vi "Toggle Output(U64).vi"(6 "Iteration Count":u64=1000, 7 "reset(F)":bool) -> (2 "Signal":bool)   [LabVIEW 2017]
doc: "Toggles the Signal output every time the iteration count reaches the configured period. Wire reset(F) to restart the toggle period."
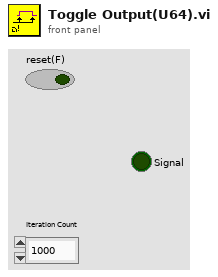
[diagram p1: front panel]
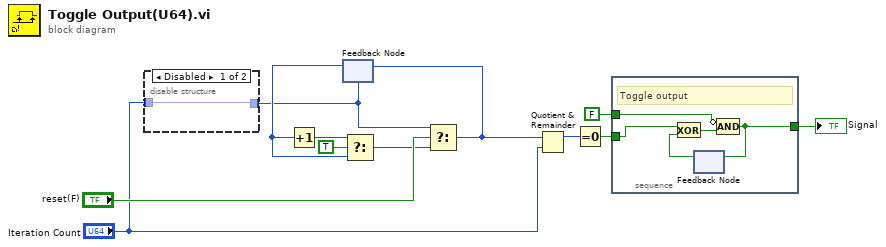
[diagram p0: block diagram]
diagram:
  n1 = disable-structure shown="Disabled" {
    disable-tunnel: "Iteration Count" -> [w13 _]
    disable-tunnel: [w13 _] -> w1
    frame Disabled {
    }
    frame Enabled {
    }
  }
  n2 = feedback #1(w1) -> (w5:u64)
  n3 = Increment(x=w5) -> (x+1=w4:u64)
  n4 = Select(t=w4, s=TRUE ("increment"), f=w5) -> (s? t:f=w3:u64)
  n5 = Select(t=w1, s="reset(F)", f=w3) -> (s? t:f=w11:u64)
  n6 = feedback-in #1(w11) -> ()
  n7 = Quotient & Remainder(x=w11, y="Iteration Count") -> (x-y*floor(x/y)=w10:u64)  [unwired: 1 out]
  n8 = Equal To 0?(x=w10) -> (x = 0?=w9:bool)
  n9 = stacked-sequence {
    tunnel: [w18] -> w8
    tunnel: FALSE ("clear") -> [w14]
    tunnel: w9 -> [w15]
    frame #0 {
      # "Toggle output"
      n10 = feedback #2() -> (w17:bool)  [unwired: 1 in]
      n11 = Exclusive Or(1:w17, 2:w15) -> (0:w16:bool)
      n12 = Compound Arithmetic op=AND(invert w14, w16) -> (w18:bool)
      n13 = feedback-in #2(w18) -> ()
    }
  }
  "Signal" <- w8
